vi "Text Description.vi"(11 "ObserverSet in":refnum<class "ObserverSet.lvclass">) -> (2 "Description":string, 3 "ObserverSet out":refnum<class "ObserverSet.lvclass">)   [LabVIEW 2011, in "Messenging.lvlib" / "ObserverSet.lvclass"]
uses:
  ObserverSet.lvclass
  SendOnly/Observer.lvclass
  Send/Send.lvclass
  Message Translation/Translator/Translator.lvclass
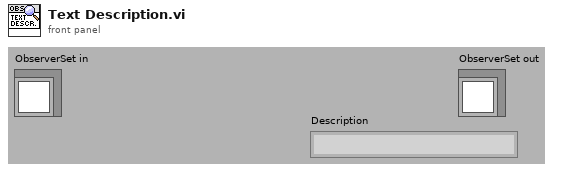
[diagram p1: front panel]
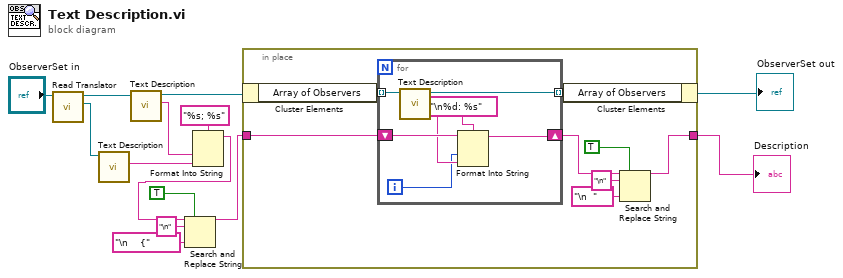
[diagram p0: block diagram]
diagram:
  n1 = call "Read Translator.vi"("Observer.lvclass in"="ObserverSet in") -> ("Messenging.lvlib:Translator.lvclass"=w9:refnum<class "Translator.lvclass">, "Observer.lvclass out"=w10:refnum<class "ObserverSet.lvclass">)  [unwired: 1 in, 8 out]
  n2 = call-dynamic "Text Description.vi"("Translator in"=w9) -> ("Description"=w7:string)  [unwired: 10 out]
  n3 = call-parent "Text Description.vi"("Send in"=w10) -> ("Description"=w6:string, "Send out"=w14:refnum<class "ObserverSet.lvclass">)  [unwired: 9 out]
  n4 = Format Into String(format string="%s; %s", w6, w7) -> (resulting string=w2:string)  [unwired: 2 in, 1 out]
  n5 = Search and Replace String(replace all?=TRUE ("replace all? (F)"), input string=w2, search string="\n", replace string="\n    {" ("replace string (\"\")")) -> (result string=w1:string)  [unwired: 1 in, 6 out]
  n6 = in-place {
    in-place-border: [w16] -> w13
    in-place-border: w1 -> [w15]
    n7 = in-place-cluster #1(w14) -> ("Array of Observers"=w22:refnum<class "Send.lvclass">[])
    n8 = for {
      tunnel: w22 -> [w29] mode=indexing
      shift-right: [w28] -> w20
      shift-left: w15 -> [w27]
      tunnel: [w25] -> w21 mode=indexing
      i -> [w23]
      n9 = call-dynamic "Text Description.vi"("Send in"=w29) -> ("Description"=w24:string, "Send out"=w25:refnum<class "Send.lvclass">)  [unwired: 9 out]
      n10 = Format Into String(format string="\n%d: %s", initial string=w27, w23, w24) -> (resulting string=w28:string)  [unwired: 1 in, 1 out]
    }
    n11 = in-place-cluster #1("Array of Observers"=w21) -> (→"ObserverSet out":refnum<class "ObserverSet.lvclass">)
    n12 = Search and Replace String(replace all?=TRUE ("replace all? (F)"), input string=w20, search string="\n", replace string="\n  " ("replace string (\"\")")) -> (result string=w16:string)  [unwired: 1 in, 6 out]
  }
  "Description" <- w13
